vi "Command - Output State.vi"(0 "VISA Refnum in":refnum<visa-resource-name>, 5 "Channel":i32, 7 "State":bool=TRUE, 11 "Error In":errorcluster) -> (4 "VISA Refnum out":refnum<visa-resource-name>, 15 "Error Out":errorcluster)   [LabVIEW 2025]
panel:
  out "Command":string
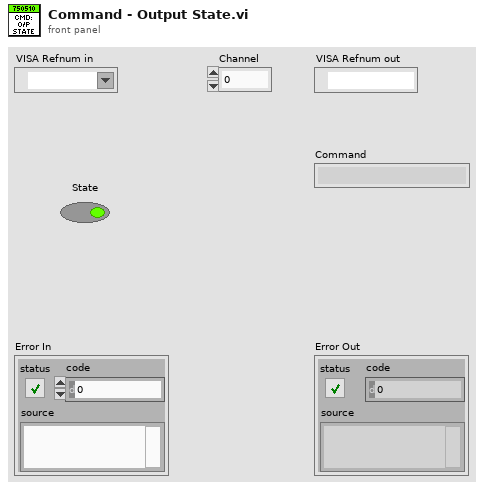
[diagram p1: front panel]
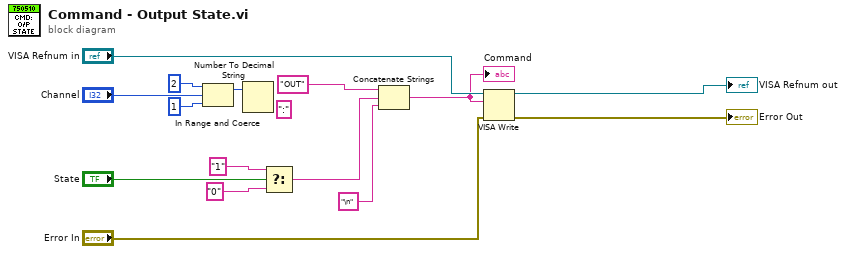
[diagram p0: block diagram]
diagram:
  (unwired) ":"
  n1 = In Range and Coerce(upper limit=2, x="Channel", lower limit=1) -> (coerced(x)=w9:i32)  [unwired: 1 out]
  n2 = Number To Decimal String(number=w9) -> ()  [unwired: 1 in, 1 out]
  n3 = Select(t="1", s="State", f="0") -> (s? t:f=w1:string)
  n4 = Concatenate Strings("OUT", w1, "\n" ("string")) -> (w11:string)
  "Command" <- w11
  n5 = VISA Write(VISA resource name="VISA Refnum in", write buffer=w11, error in (no error)="Error In") -> (VISA resource name out=→"VISA Refnum out":refnum<visa-resource-name>, error out=→"Error Out":errorcluster)  [unwired: 1 out]
